vi "random_name.vi"() -> ()   [LabVIEW 2015]
uses:
  <vilib>/Utility/file.llb/Read Delimited Spreadsheet (string).vi
  <vilib>/Analysis/1siggen.llb/Riffle Array (I32).vi
  <vilib>/Analysis/NI_AALBase.lvlib
panel:
  in  "File Path":path
  in  "Save Button":bool
  in  "Exit Program":bool
  in  "Proceed Button":bool
  in  "Single row                      or                 multiple rows":bool
  in  "single row to use":dbl
  in  "rows to concatenate (comma delimindated)":string
  in  "which elements do you want to delete (comma deliminated)":string
  out "Group Array":string[](array[string])
  in  "group size":dbl
  out "all rows":string[][](array[string])
  # "Step 1: View the Input file"
  # "Step 2: Choose which rows will be input"
  # "Step 3: Decide if you need to delete elements and establish group size"
  # "Results"
  # "Step 4: Proceed"
  # "Step 5: Save or Exit"
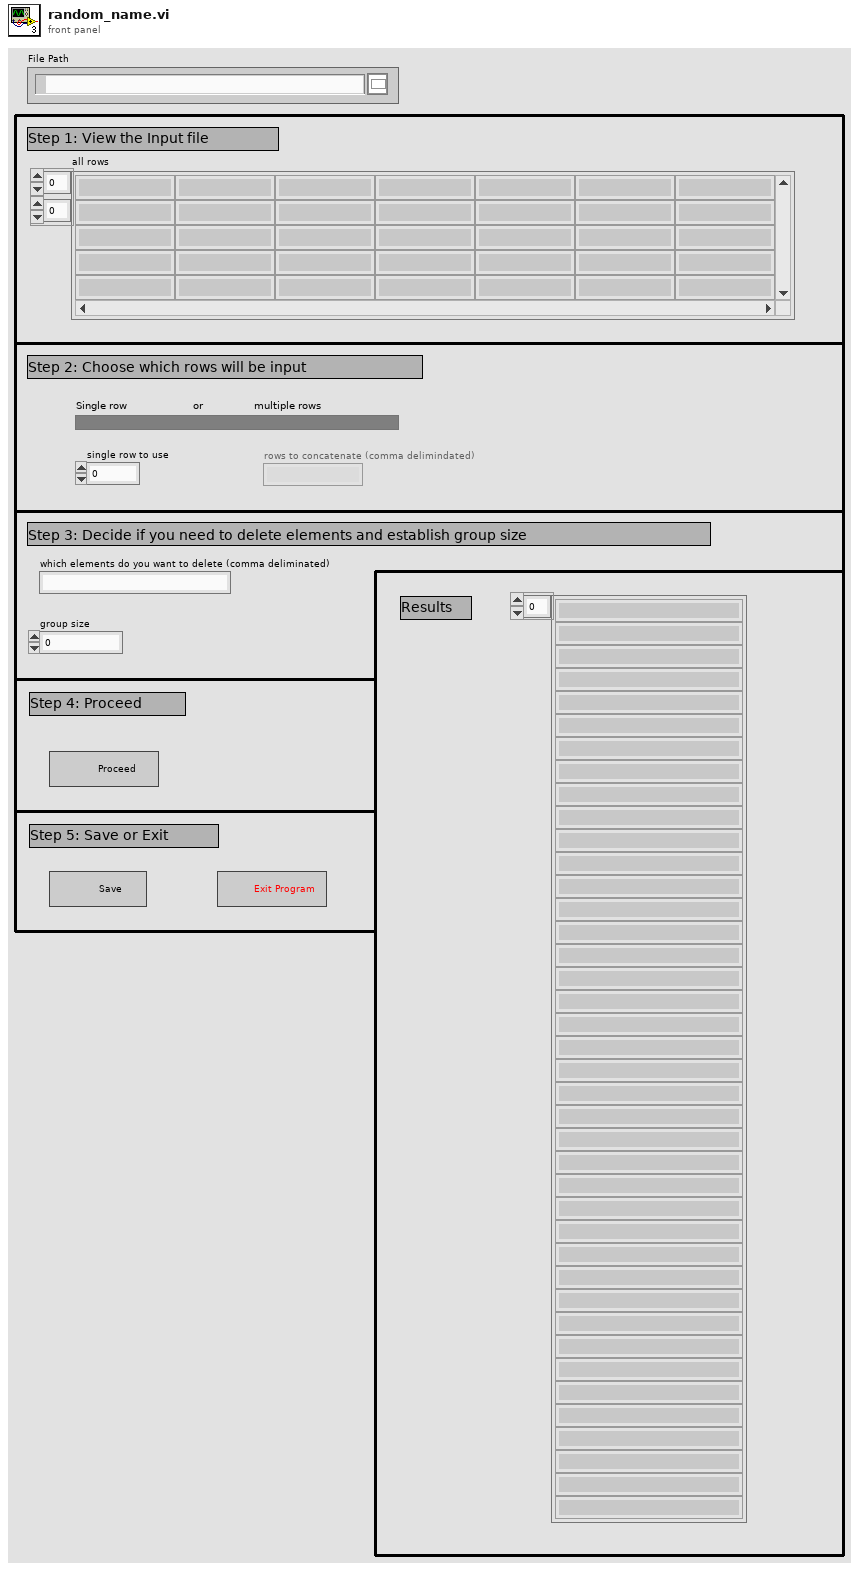
[diagram p1: front panel]
types:
  T1 = enum8{"Enabled", "Disabled", "Disabled and Grayed Out"}
  T2 = enum16{"open", "replace", "create", "open or create", "replace or create", "replace or create with confirmation"}
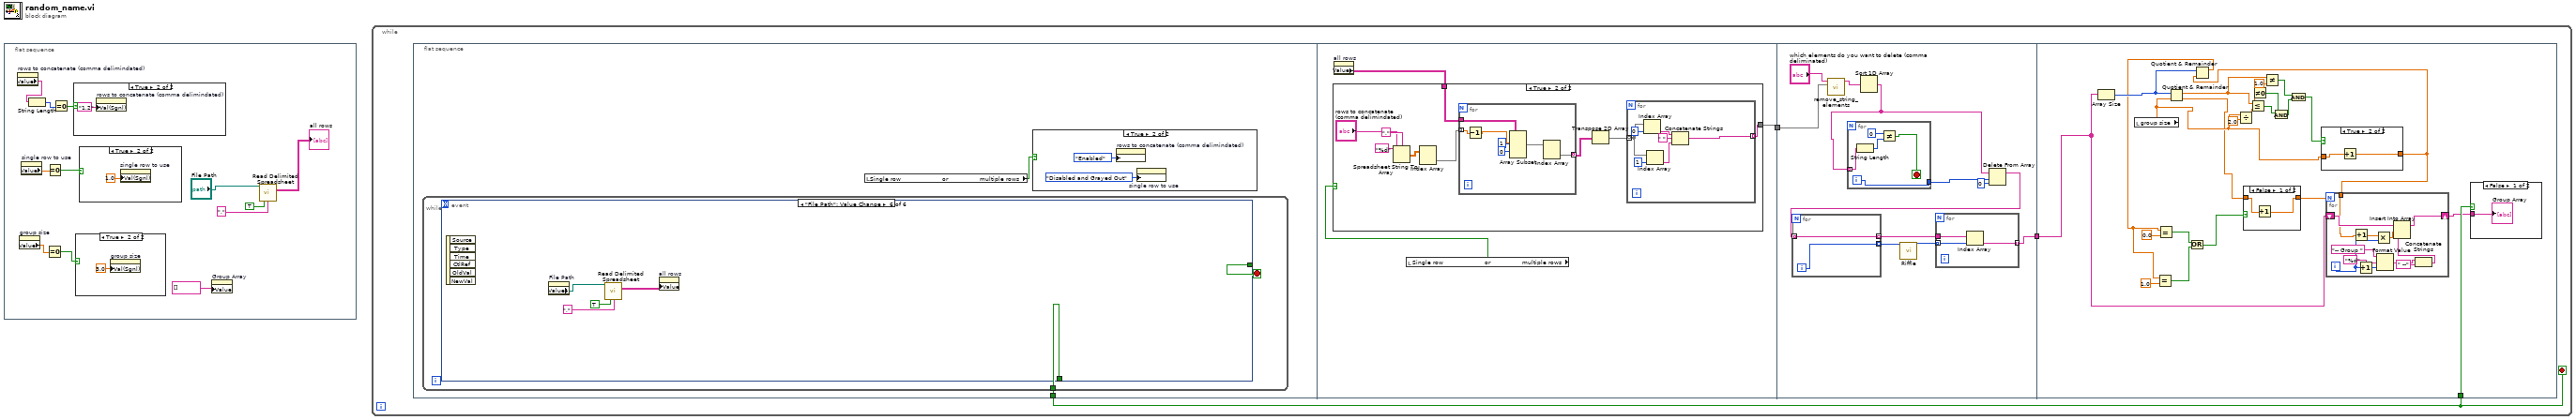
[diagram p0: block diagram]
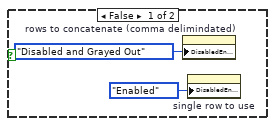
[diagram p2: hidden frame]
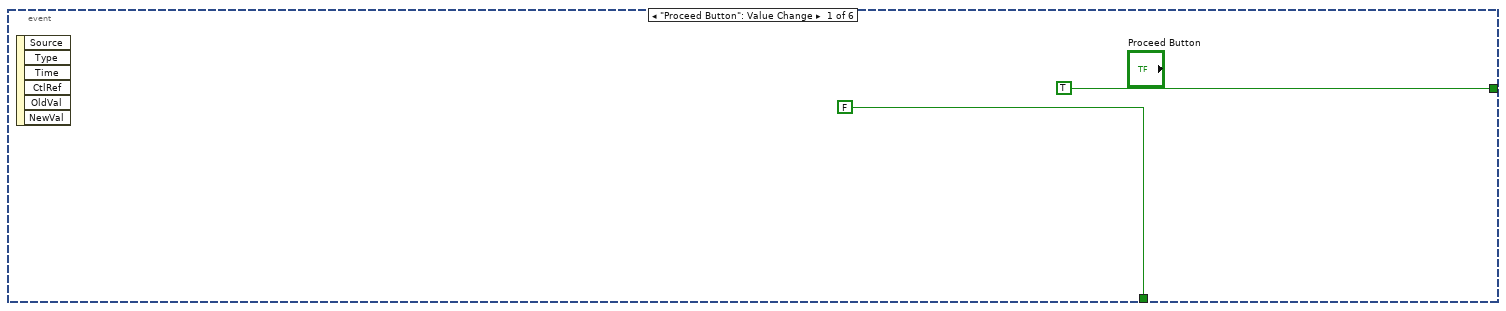
[diagram p3: hidden frame]
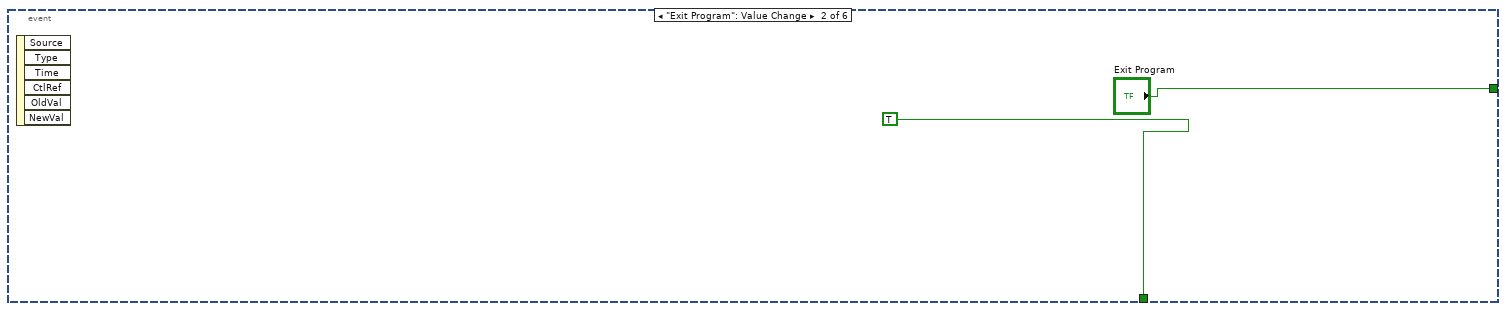
[diagram p4: hidden frame]
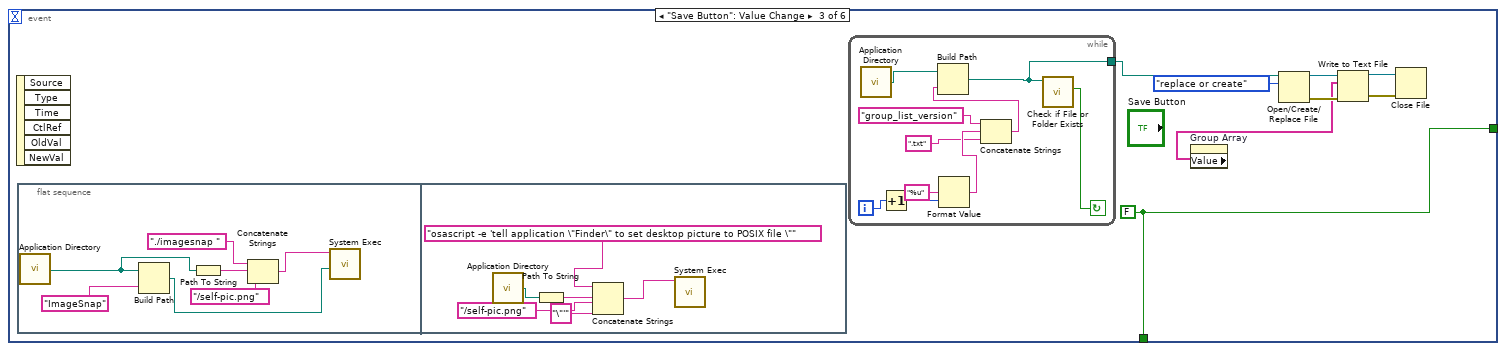
[diagram p5: hidden frame]
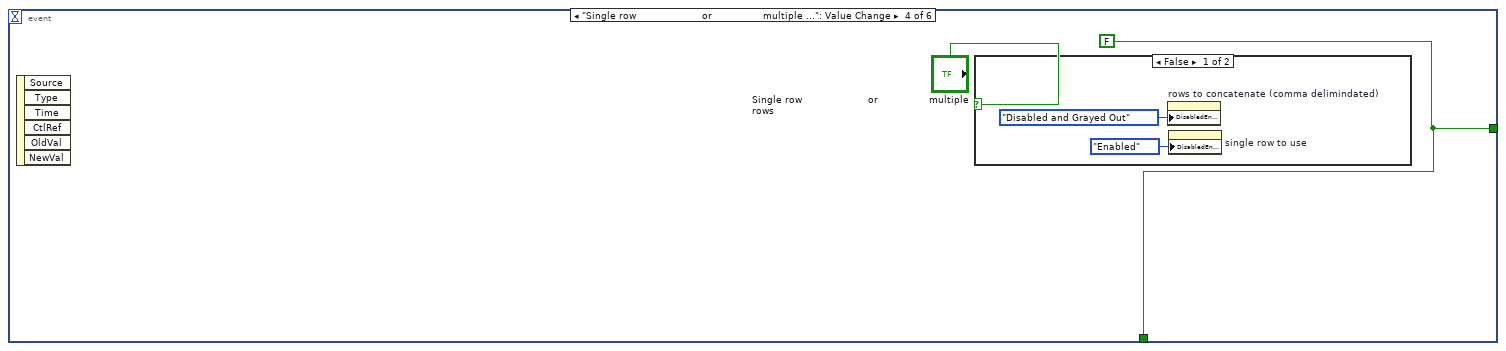
[diagram p6: hidden frame]
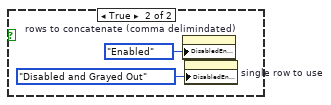
[diagram p7: hidden frame]
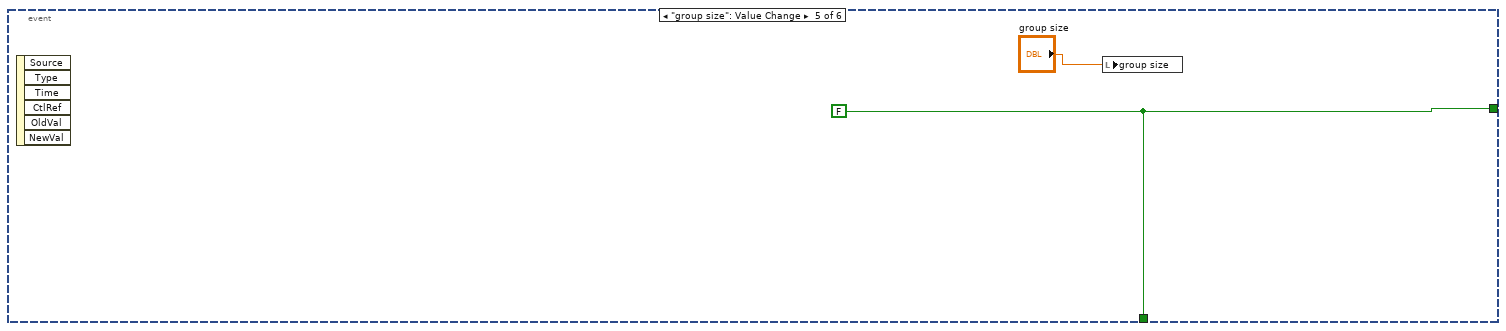
[diagram p8: hidden frame]
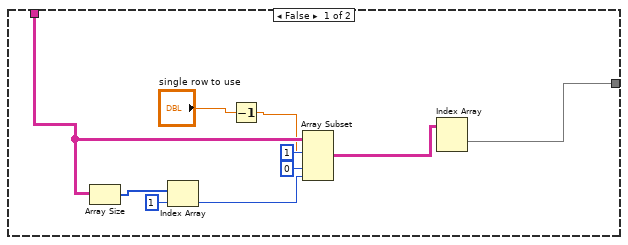
[diagram p9: hidden frame]
diagram:
  n1 = flat-sequence {
    frame #0 {
      n2 = property on="rows to concatenate (comma delimindated)" class="Str"() -> ("Value"=w10:string)  [unwired: 2 in, 2 out]
      n3 = property on="group size" class="DigNum (strict)"() -> ("Value"=w6:dbl)  [unwired: 2 in, 2 out]
      n4 = property on="single row to use" class="DigNum (strict)"() -> ("Value"=w8:dbl)  [unwired: 2 in, 2 out]
      n5 = String Length(string=w10) -> (length=w11:i32)
      n6 = Equal To 0?(x=w6) -> (x = 0?=w7:bool)
      n7 = Equal To 0?(x=w8) -> (x = 0?=w9:bool)
      n8 = Equal To 0?(x=w11) -> (x = 0?=w12:bool)
      n9 = case shown="True" w12 {
        frame False {
        }
        frame True {
          n10 = property on="rows to concatenate (comma delimindated)" class="Str"("Val(Sgnl)"="1,2" ("Value (Signaling)")) -> ()  [unwired: 2 in, 2 out]
        }
      }
      n11 = case shown="True" w7 {
        frame False {
        }
        frame True {
          n12 = property on="group size" class="DigNum (strict)"("Val(Sgnl)"=3.0 ("Value (Signaling)")) -> ()  [unwired: 2 in, 2 out]
        }
      }
      n13 = case shown="True" w9 {
        frame False {
        }
        frame True {
          n14 = property on="single row to use" class="DigNum (strict)"("Val(Sgnl)"=1.0 ("Value (Signaling)")) -> ()  [unwired: 2 in, 2 out]
        }
      }
      n15 = property on="Group Array" class="Arr (strict)"("Value"=string[] []) -> ()  [unwired: 2 in, 2 out]
      n16 = call-poly <vilib>:"Read Delimited Spreadsheet.vi"("file path (dialog if empty)"="File Path", "transpose? (F)"=TRUE, "delimiter (\\t)"="," ("delimiter (\\t)")) -> ("all rows"=→"all rows":string[][])  [unwired: 7 in, 5 out]
    }
  }
  n17 = while {
    stop <- w16 stop-if-true
    n18 = flat-sequence {
      tunnel: [w19] -> w16
      tunnel: [w76] -> w18
      tunnel: w18 -> [w120]
      tunnel: [w110] -> w17
      tunnel: w17 -> [w134]
      tunnel: w16 -> [w132]
      frame #0 {
        n19 = while {
          tunnel: [w25] -> w19
          stop <- w26 stop-if-true
          n20 = event shown="[5] \"File Path\": Value Change" {
            selector: _ -> [_ _ _ _ _ _]
            dyn-events: _ -> [_ _ _ _ _ _]
            timeout: _ -> [_ _ _ _ _ _]
            tunnel: [TRUE "Exit Program" w31 w62 w68 _] -> w26
            tunnel: [FALSE TRUE w31 w62 w68 _] -> w25
            event "Proceed Button": Value Change {
              n21 = event-data() -> ()  [unwired: 1 in, 6 out]
            }
            event "Exit Program": Value Change {
              n22 = event-data() -> ()  [unwired: 1 in, 6 out]
            }
            event "Save Button": Value Change {
              w31 = FALSE
              n23 = event-data() -> ()  [unwired: 1 in, 6 out]
              n24 = flat-sequence {
                frame #0 {
                  n25 = call <vilib>:"Application Directory.vi"() -> ("Application Directory"=w45:path)
                  n26 = Build Path(base path=w45, name or relative path="ImageSnap") -> (appended path=w40:path)
                  n27 = Path To String(path=w45) -> (string=w41:string)
                  n28 = Concatenate Strings("./imagesnap " ("command line"), w41, "/self-pic.png") -> (w43:string)
                  n29 = call <vilib>:"System Exec.vi"("working directory"=w40, "command line"=w43) -> ()  [unwired: 6 in, 4 out]
                }
                frame #1 {
                  n30 = call <vilib>:"Application Directory.vi"() -> ("Application Directory"=w47:path)
                  n31 = Path To String(path=w47) -> (string=w49:string)
                  n32 = Concatenate Strings("osascript -e 'tell application \"Finder\" to set desktop picture to POSIX file \"" ("command line"), w49, "/self-pic.png", "\"'" ("string")) -> (w51:string)
                  n33 = call <vilib>:"System Exec.vi"("command line"=w51) -> ()  [unwired: 7 in, 4 out]
                }
              }
              n34 = while {
                tunnel: [w53] -> w34
                i -> [w60]
                stop <- w54 continue-if-true
                n35 = call <vilib>:"Application Directory.vi"() -> ("Application Directory"=w61:path)
                n36 = Increment(x=w60) -> (x+1=w59:i32)
                n37 = Format Value(format string="%u", value (0)=w59) -> (output string=w58:string)  [unwired: 1 in]
                n38 = Concatenate Strings("group_list_version", w58, ".txt") -> (w55:string)
                n39 = Build Path(base path=w61, name or relative path=w55) -> (appended path=w53:path)
                n40 = call <vilib>:"Check if File or Folder Exists.vi"("path"=w53) -> ("file or folder exists?"=w54:bool)  [unwired: 8 in, 2 out]
              }
              n41 = property on="Group Array" class="Arr (strict)"() -> ("Value"=w32:string[])  [unwired: 2 in, 2 out]
              n42 = Open/Create/Replace File(file path (use dialog)=w34, operation (0:open)=T2."replace or create") -> (refnum out=w38:refnum<file>, error out=w35:errorcluster)  [unwired: 4 in, 1 out]
              n43 = Write to Text File(file (use dialog)=w38, text=w32, error in=w35) -> (refnum out=w37:refnum<file>, error out=w36:errorcluster)  [unwired: 1 in, 1 out]
              n44 = Close File(refnum=w37, error in=w36) -> ()  [unwired: 2 out]
            }
            event "Single row                      or                 multiple rows": Value Change {
              w62 = FALSE
              n45 = event-data() -> ()  [unwired: 1 in, 6 out]
              n46 = case shown="False" "Single row                      or                 multiple rows" {
                frame False {
                  n47 = property on="rows to concatenate (comma delimindated)" class="Str"("DisabledEnum"=T1."Disabled and Grayed Out" ("Disabled")) -> ()  [unwired: 2 in, 2 out]
                  n48 = property on="single row to use" class="DigNum (strict)"("DisabledEnum"=T1."Enabled" ("Disabled")) -> ()  [unwired: 2 in, 2 out]
                }
                frame True {
                  n49 = property on="rows to concatenate (comma delimindated)" class="Str"("DisabledEnum"=T1."Enabled" ("Disabled")) -> ()  [unwired: 2 in, 2 out]
                  n50 = property on="single row to use" class="DigNum (strict)"("DisabledEnum"=T1."Disabled and Grayed Out" ("Disabled")) -> ()  [unwired: 2 in, 2 out]
                }
              }
            }
            event "group size": Value Change {
              w68 = FALSE
              n51 = event-data() -> ()  [unwired: 1 in, 6 out]
              n52 = local write "group size"("group size") -> ()
            }
            event "File Path": Value Change {
              n53 = event-data() -> ()  [unwired: 1 in, 6 out]
              n54 = property on="File Path" class="Path"() -> ("Value"=w71:path)  [unwired: 2 in, 2 out]
              n55 = call-poly <vilib>:"Read Delimited Spreadsheet.vi"("file path (dialog if empty)"=w71, "transpose? (F)"=TRUE, "delimiter (\\t)"="," ("delimiter (\\t)")) -> ("all rows"=w70:string[][])  [unwired: 7 in, 5 out]
              n56 = property on="all rows" class="Arr (strict)"("Value"=w70) -> ()  [unwired: 2 in, 2 out]
            }
          }
        }
        n57 = local read "Single row                      or                 multiple rows"() -> (w20:bool)
        n58 = case shown="True" w20 {
          frame False {
            n59 = property on="rows to concatenate (comma delimindated)" class="Str"("DisabledEnum"=T1."Disabled and Grayed Out" ("Disabled")) -> ()  [unwired: 2 in, 2 out]
            n60 = property on="single row to use" class="DigNum (strict)"("DisabledEnum"=T1."Enabled" ("Disabled")) -> ()  [unwired: 2 in, 2 out]
          }
          frame True {
            n61 = property on="rows to concatenate (comma delimindated)" class="Str"("DisabledEnum"=T1."Enabled" ("Disabled")) -> ()  [unwired: 2 in, 2 out]
            n62 = property on="single row to use" class="DigNum (strict)"("DisabledEnum"=T1."Disabled and Grayed Out" ("Disabled")) -> ()  [unwired: 2 in, 2 out]
          }
        }
      }
      frame #1 {
        n63 = property on="all rows" class="Arr (strict)"() -> ("Value"=w74:string[][])  [unwired: 2 in, 2 out]
        n64 = local read "Single row                      or                 multiple rows"() -> (w75:bool)
        n65 = case shown="True" w75 {
          tunnel: w74 -> [w81 w93]
          tunnel: [w79 w92] -> w76
          frame False {
            n66 = Array Size(array=w81) -> (size(s)=w86:i32[])
            n67 = Index Array(array=w86, index=1) -> (element=w84:i32)
            n68 = Decrement(x="single row to use") -> (x-1=w77:dbl)
            n69 = Array Subset(array=w81, index (row)=w77, length (row)=1 ("length"), index (col)=0 ("index"), length (col)=w84) -> (w80:string[][])
            n70 = Index Array(array=w80) -> (element=w79:string[])  [unwired: 2 in]
          }
          frame True {
            n71 = Spreadsheet String To Array(delimiter (Tab)=",", format string="%d", spreadsheet string="rows to concatenate (comma delimindated)") -> (array=w88:dbl[][])  [unwired: 1 in]
            n72 = Index Array(array=w88) -> (element=w87:dbl[])  [unwired: 2 in]
            n73 = for {
              tunnel: w87 -> [w103] mode=indexing
              tunnel: w93 -> [w107]
              tunnel: [w105] -> w94 mode=indexing
              n74 = Decrement(x=w103) -> (x-1=w104:dbl)
              n75 = Array Subset(array=w107, index (row)=w104, length (row)=1 ("length"), index (col)=0 ("index")) -> (w106:string[][])  [unwired: 1 in]
              n76 = Index Array(array=w106) -> (element=w105:string[])  [unwired: 2 in]
            }
            n77 = Transpose 2D Array(2D array=w94) -> (transposed array=w95:string[][])
            n78 = for {
              tunnel: w95 -> [w102] mode=indexing
              tunnel: [w98] -> w92 mode=indexing
              n79 = Index Array(array=w102, index=0) -> (element=w99:string)
              n80 = Index Array(array=w102, index=1) -> (element=w97:string)
              n81 = Concatenate Strings(w99, " " ("string"), w97) -> (w98:string)
            }
          }
        }
      }
      frame #2 {
        n82 = call "remove_string_elements.vi"("Array in"=w120, "spreadsheet string"="which elements do you want to delete (comma deliminated)") -> ("Array out"=w118:string[])  [unwired: 9 in]
        n83 = Sort 1D Array(array=w118) -> (sorted array=w115:string[])
        n84 = for {
          tunnel: w115 -> [w128] mode=indexing
          tunnel: [w126] -> w116
          i -> [w126]
          stop <- w127 stop-if-true
          n85 = String Length(string=w128) -> (length=w130:i32)
          n86 = Not Equal?(x=0, y=w130) -> (x != y?=w127:bool)
        }
        n87 = Delete From Array(array=w115, length=w116, index=0) -> (array with subset deleted=w114:string[])  [unwired: 1 out]
        n88 = for {
          tunnel: [w125] -> w113 mode=indexing
          tunnel: w114 -> [w124] mode=indexing
          tunnel: [w124] -> w112 mode=indexing
          i -> [w125]
        }
        n89 = call-poly <vilib>:"Riffle.vi"("X"=w113) -> ("Riffled {X}"=w111:i32[])  [unwired: 8 in, 2 out]
        n90 = for {
          tunnel: w111 -> [w123] mode=indexing
          tunnel: w112 -> [w122]
          tunnel: [w121] -> w110 mode=indexing
          n91 = Index Array(array=w122, index=w123) -> (element=w121:string)
        }
      }
      frame #3 {
        n92 = Array Size(array=w134) -> (size(s)=w142:i32)
        n93 = local read "group size"() -> (w148:dbl)
        n94 = Quotient & Remainder(x=w142, y=w148) -> (x-y*floor(x/y)=w153:dbl, floor(x/y)=w140:dbl)
        n95 = Divide(x=w148, y=2.0) -> (x/y=w145:dbl)
        n96 = Less Or Equal?(x=w153, y=w145) -> (x <= y?=w147:bool)
        n97 = Not Equal To 0?(x=w153) -> (x != 0?=w146:bool)
        n98 = Not Equal?(x=w153, y=1.0) -> (x != y?=w150:bool)
        n99 = And(x=w147, y=w146) -> (x .and. y?=w151:bool)
        n100 = And(x=w150, y=w151) -> (x .and. y?=w152:bool)
        n101 = case shown="True" w152 {
          tunnel: w148 -> [w155 w157]
          tunnel: [w155 w156] -> w143
          frame False {
          }
          frame True {
            n102 = Increment(x=w157) -> (x+1=w156:dbl)
          }
        }
        n103 = Quotient & Remainder(x=w142, y=w143) -> (x-y*floor(x/y)=w141:dbl)  [unwired: 1 out]
        n104 = Equal?(x=w141, y=1.0) -> (x = y?=w138:bool)
        n105 = Equal?(x=w141, y=0.0) -> (x = y?=w137:bool)
        n106 = Or(x=w137, y=w138) -> (x .or. y?=w139:bool)
        n107 = case shown="False" w139 {
          tunnel: w140 -> [w159 w160]
          tunnel: [w158 w160] -> w133
          frame False {
            n108 = Increment(x=w159) -> (x+1=w158:dbl)
          }
          frame True {
          }
        }
        n109 = for {
          N: w133 -> [_]
          tunnel: w143 -> [w167]
          shift-right: [w170] -> w131
          shift-left: w134 -> [w169]
          i -> [w165]
          n110 = Increment(x=w167) -> (x+1=w166:dbl)
          n111 = Increment(x=w165) -> (x+1=w164:i32)
          n112 = Multiply(x=w166, y=w165) -> (x*y=w172:dbl)
          n113 = Format Value(string ("")="-- Group ", format string="%d", value (0)=w164) -> (output string=w162:string)
          n114 = Concatenate Strings(w162, " --" ("string")) -> (w163:string)
          n115 = Insert Into Array(array=w169, index=w172, new element=w163) -> (w170:string[])
        }
        n116 = case shown="False" w132 {
          tunnel: w131 -> [w154 _]
          frame False {
            "Group Array" <- w154
          }
          frame True {
          }
        }
      }
    }
  }
